vi "UI-EnqueueCmd.vi"(8 "error in (no error)":errorcluster, 9 "Data":variant, 10 "Cmd":T1, 11 "Queue In":refnum<queue>) -> (0 "error out":errorcluster, 3 "Queue Out":refnum<queue>)   [LabVIEW 2024, in "Scripts.lvlib"]
uses:
  Scripts.lvlib
  UI-Cmd--enum.ctl
  UI-Cmd--cluster.ctl
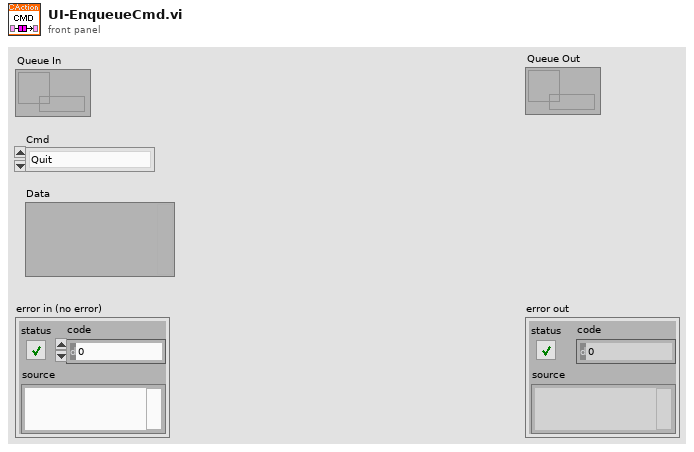
[diagram p1: front panel]
types:
  T1 = typedef "Scripts.lvlib/UI-Cmd--enum.ctl" = enum16{"Quit"}
  T2 = typedef "Scripts.lvlib/UI-Cmd--cluster.ctl" = cluster{"Cmd":T1, "Data":variant}
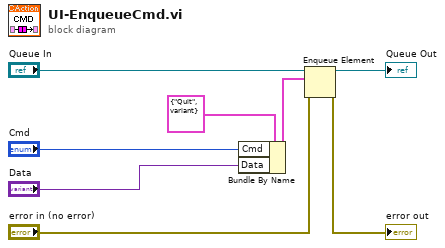
[diagram p0: block diagram]
diagram:
  n1 = Bundle By Name(cluster=T2 {"Cmd"=enum."Quit", "Data"=variant} ("element"), "Cmd"="Cmd", "Data"="Data") -> (w3:T2)
  n2 = Enqueue Element(queue="Queue In", element=w3, error in (no error)="error in (no error)") -> (queue out=→"Queue Out":refnum<queue>, error out=→"error out":errorcluster)  [unwired: 1 in, 1 out]
